vi "Rotation_Plus.vi"(9 "other ROTATION":T1, 11 "in ROTATION":T1) -> (3 "out ROTATION":T1)   [LabVIEW 2019, in "PathExecution_Library.lvlib"]
uses:
  PathExecution_Library.lvlib
  ROTATION.ctl
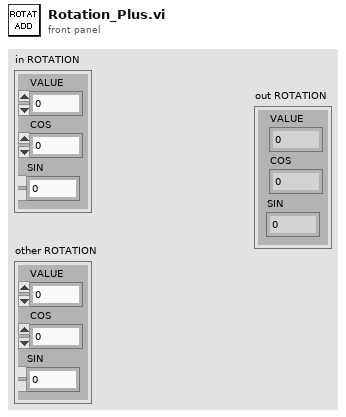
[diagram p1: front panel]
types:
  T1 = typedef "PathExecution_Library.lvlib/ROTATION.ctl" = cluster{"VALUE":dbl, "COS":dbl, "SIN":dbl}
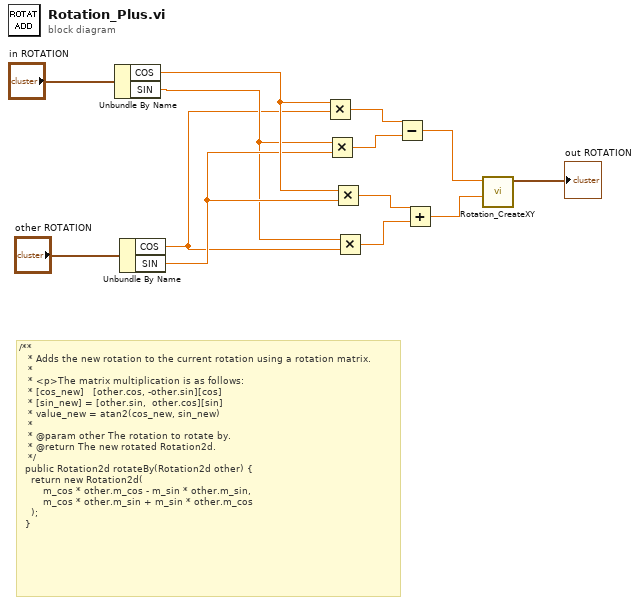
[diagram p0: block diagram]
diagram:
  # "/**\n   * Adds the new rotation to the current rotation using a rotation matrix.\n   *\n   * <p>The matrix multiplication is as follows:\n   * [cos_new]   [other.cos, -other.sin][cos]\n   * [sin_new] = [other.sin,  other.cos][sin]\n   * value_new = atan2(cos_new, sin_new)\n   *\n   * @param other The rotation to rotate by.\n   * @return The new rotated Rotation2d.\n   */\n  public Rotation2d rotateBy(Rotation2d other) {\n    return new Rotation2d(\n        m_cos * other.m_cos - m_sin * other.m_sin,\n        m_cos * other.m_sin + m_sin * other.m_cos\n    );\n  }"
  n1 = Unbundle By Name("in ROTATION") -> ("COS"=w5:dbl, "SIN"=w3:dbl)
  n2 = Unbundle By Name("other ROTATION") -> ("COS"=w2:dbl, "SIN"=w4:dbl)
  n3 = Multiply(x=w5, y=w2) -> (x*y=w11:dbl)
  n4 = Multiply(x=w3, y=w4) -> (x*y=w10:dbl)
  n5 = Multiply(x=w5, y=w4) -> (x*y=w7:dbl)
  n6 = Multiply(x=w3, y=w2) -> (x*y=w6:dbl)
  n7 = Subtract(x=w11, y=w10) -> (x-y=w8:dbl)
  n8 = Add(x=w7, y=w6) -> (x+y=w1:dbl)
  n9 = call "Rotation_CreateXY.vi"("Y or sine"=w1, "X or  cosine"=w8) -> ("ROTATION"=→"out ROTATION":T1)  [unwired: 9 in]
